vi "Add Seq.vi"(8 "error in (no error)":errorcluster, 11 "[V]System Tree View in":refnum<class "[V]System Tree View.lvclass">) -> (0 "error out":errorcluster, 3 "[V]System Tree View out":refnum<class "[V]System Tree View.lvclass">)   [LabVIEW 2020]
uses:
  <vilib>/HUASUI/Tree/Item/Type Definitions/Item Map.ctl
  <vilib>/HUASUI/Tree/Item/Item.lvclass
  <vilib>/HUASUI/Tree/Tree Helper/Tree Helper.lvclass
  <vilib>/HUASUI/Tree/Tree Helper.lvlib
  [V]System Tree View.lvclass
  C:/Program Files (x86)/National Instruments/LabVIEW 2020/vi.lib/ActorFramework/Actor/Actor.lvclass
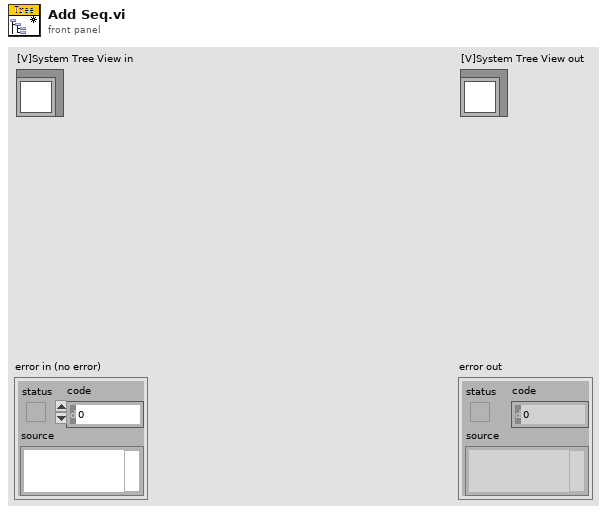
[diagram p1: front panel]
types:
  T1 = typedef "Tree Helper.lvlib/Item.lvclass/Item Map.ctl" = cluster{"Self Tag":string, "Parent Tag":string, "LeftCell Value":string, "RightCells Value":string[], "Is Child":bool, "Symbol Index":i32}
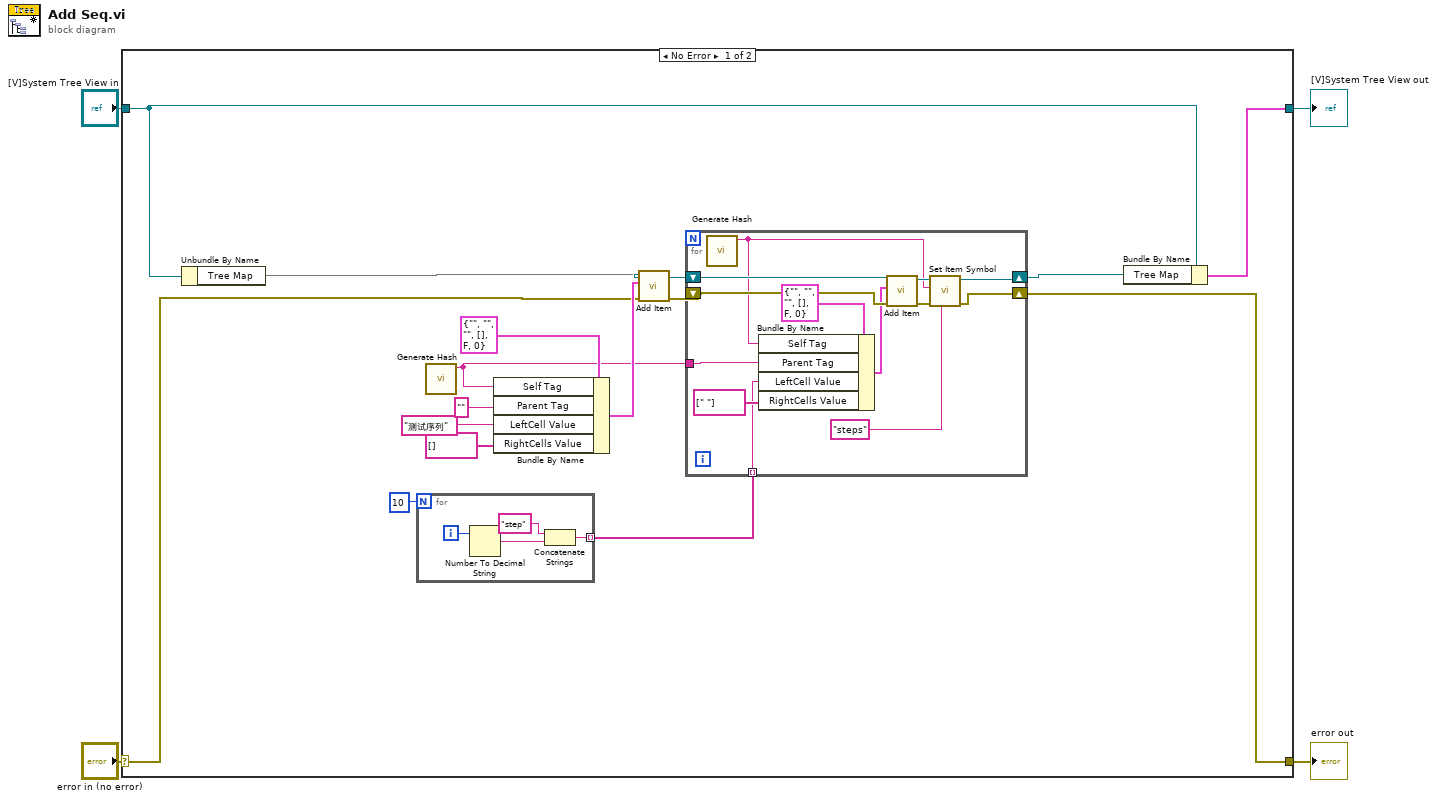
[diagram p0: block diagram]
diagram:
  n1 = case shown="No Error" "error in (no error)" {
    selector: "error in (no error)" -> [w8 w39]
    tunnel: [w6 w39] -> w3
    tunnel: [w5 w38] -> w1
    tunnel: "[V]System Tree View in" -> [w7 w38]
    frame No Error {
      n2 = Unbundle By Name(w7) -> ("Tree Map"=w12)
      n3 = for {
        N: 10 -> [_]
        tunnel: [w21] -> w10 mode=indexing
        i -> [w22]
        n4 = Number To Decimal String(number=w22) -> (decimal integer string=w23:string)  [unwired: 1 in]
        n5 = Concatenate Strings("step" ("string"), w23) -> (w21:string)
      }
      n6 = call <vilib>:"Generate Hash.vi"() -> ("Hash"=w13:string)  [unwired: 10 in, 1 out]
      n7 = Bundle By Name(cluster=T1 {"Self Tag"="", "Parent Tag"="", "LeftCell Value"="", "RightCells Value"=[], "Is Child"=FALSE, "Symbol Index"=0} ("Item Map"), "Self Tag"=w13, "Parent Tag"="", "LeftCell Value"="测试序列", "RightCells Value"=string[] []) -> (w17:T1)
      n8 = call <vilib>:"Add Item.vi"("error in (no error)"=w8, "Item Map"=w17, "Tree Map in"=w12) -> ("error out"=w19:errorcluster, "Tree Map out"=w20:refnum<class "Tree Helper.lvclass">)  [unwired: 7 in]
      n9 = for {
        shift-right: [w35] -> w9
        shift-left: w20 -> [w36]
        tunnel: w10 -> [w33] mode=indexing
        shift-right: [w31] -> w6
        shift-left: w19 -> [w30]
        tunnel: w13 -> [w29]
        n10 = call <vilib>:"Generate Hash.vi"() -> ("Hash"=w28:string)  [unwired: 10 in, 1 out]
        n11 = Bundle By Name(cluster=T1 {"Self Tag"="", "Parent Tag"="", "LeftCell Value"="", "RightCells Value"=[], "Is Child"=FALSE, "Symbol Index"=0} ("Item Map"), "Self Tag"=w28, "Parent Tag"=w29, "LeftCell Value"=w33, "RightCells Value"=string[] [" "]) -> (w25:T1)
        n12 = call <vilib>:"Add Item.vi"("error in (no error)"=w30, "Item Map"=w25, "Tree Map in"=w36) -> ("error out"=w27:errorcluster, "Tree Map out"=w37:refnum<class "Tree Helper.lvclass">)  [unwired: 7 in]
        n13 = call <vilib>:"Set Item Symbol.vi"("IconName"="steps", "error in (no error)"=w27, "Tag"=w28, "Tree Map in"=w37) -> ("error out"=w31:errorcluster, "Tree Map out"=w35:refnum<class "Tree Helper.lvclass">)  [unwired: 6 in]
      }
      n14 = Bundle By Name(cluster=w7, "Tree Map"=w9) -> (w5:cluster{})
    }
    frame Error {
    }
  }
  "error out" <- w3
  "[V]System Tree View out" <- w1
